vi "RevSecToVelo.vi"(1 "Revolutions/s":dbl) -> (0 "Velocity":dbl)   [LabVIEW 2014]
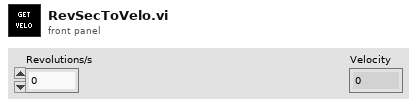
[diagram p1: front panel]
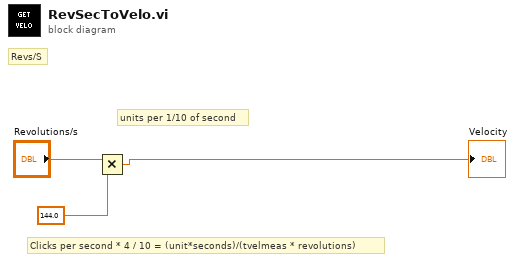
[diagram p0: block diagram]
diagram:
  # "Clicks per second * 4 / 10 = (unit*seconds)/(tvelmeas * revolutions)"
  # "Revs/S"
  # "units per 1/10 of second"
  n1 = Multiply(x="Revolutions/s", y=144.0) -> (x*y=→"Velocity":dbl)
